vi "Flock_Master_WriteNewRev.vi"(0 "configuration file path":path=path "C:/Users/mblack/test/mblack-harrypotter2-test/user/mblack/FRC Team Service/Trunk/2.0/Master/source/Static Source/master/FRCts.ini", 1 "MajorRev":i32=2, 2 "MinorRev":i32, 4 "BuildNum":i32, 5 "error in (no error)":errorcluster, 6 "IterationNum":i32) -> (19 "error out":errorcluster)   [LabVIEW 2014, in "FA_Agent_BuildRevision.lvlib"]
uses:
  FA_Agent_BuildRevision.lvlib
  <vilib>/Utility/config.llb/Write Key (I32).vi
  <vilib>/Utility/config.llb/NI_LVConfig.lvlib
panel:
  in  "create file if necessary (T)":bool=TRUE
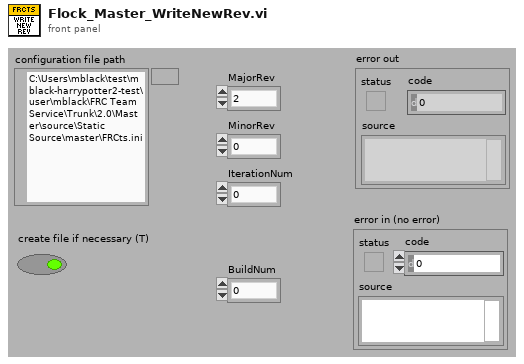
[diagram p1: front panel]
types:
  T1 = typedef "NI_LVConfig.lvlib/Config Data RefNum.ctl" = refnum<k1>
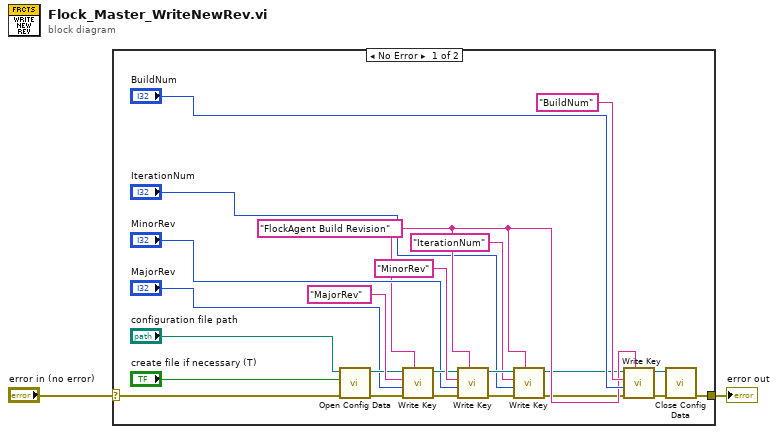
[diagram p0: block diagram]
diagram:
  n1 = case shown="No Error" "error in (no error)" {
    selector: "error in (no error)" -> [w10 w26]
    tunnel: [w12 w26] -> w2
    frame No Error {
      w8 = "FlockAgent Build Revision"
      n2 = call <vilib>:"Open Config Data.vi"("error in (no error)"=w10, "create file if necessary (T)"="create file if necessary (T)", "configuration file path"="configuration file path") -> ("error out"=w20:errorcluster, "refnum"=w19:T1)  [unwired: 6 in, 1 out]
      n3 = call-poly <vilib>:"Write Key.vi"("section"=w8, "error in (no error)"=w20, "value"="MajorRev", "key"="MajorRev", "refnum"=w19) -> ("error out"=w23:errorcluster, "refnum out"=w22:T1)  [unwired: 4 in, 1 out]
      n4 = call-poly <vilib>:"Write Key.vi"("section"=w8, "error in (no error)"=w23, "value"="MinorRev", "key"="MinorRev", "refnum"=w22) -> ("error out"=w7:errorcluster, "refnum out"=w9:T1)  [unwired: 4 in, 1 out]
      n5 = call-poly <vilib>:"Write Key.vi"("section"=w8, "error in (no error)"=w7, "value"="IterationNum", "key"="IterationNum", "refnum"=w9) -> ("error out"=w3:errorcluster, "refnum out"=w4:T1)  [unwired: 4 in, 1 out]
      n6 = call-poly <vilib>:"Write Key.vi"("section"=w8, "error in (no error)"=w3, "value"="BuildNum", "key"="BuildNum", "refnum"=w4) -> ("error out"=w13:errorcluster, "refnum out"=w11:T1)  [unwired: 4 in, 1 out]
      n7 = call <vilib>:"Close Config Data.vi"("error in (no error)"=w13, "refnum"=w11) -> ("error out"=w12:errorcluster)  [unwired: 8 in, 1 out]
    }
    frame Error {
    }
  }
  "error out" <- w2
